vi "Configure Temperature Setpoint.vi"(8 "error in (no error)":errorcluster, 10 "Stirrer Speed Setpoint":dbl, 11 "heater_explorer in":refnum<class "heater_explorer.lvclass">) -> (0 "error out":errorcluster, 3 "heater_explorer out":refnum<class "heater_explorer.lvclass">)   [LabVIEW 2020, in "polar_bear_plus_drivers.lvlib" / "heater_explorer.lvclass"]
doc: "Changes the temperature setpoint."
uses:
  <instrlib>/RxnRover/Driver Polar Bear Plus/heater_explorer/heater_explorer.lvclass
  <instrlib>/RxnRover/Driver Polar Bear Plus/heater_explorer/heater_explorer.lvclass/heater_explorer.ctl
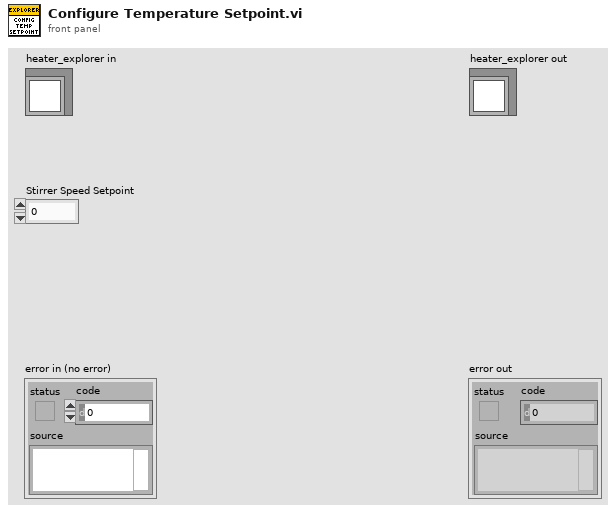
[diagram p1: front panel]
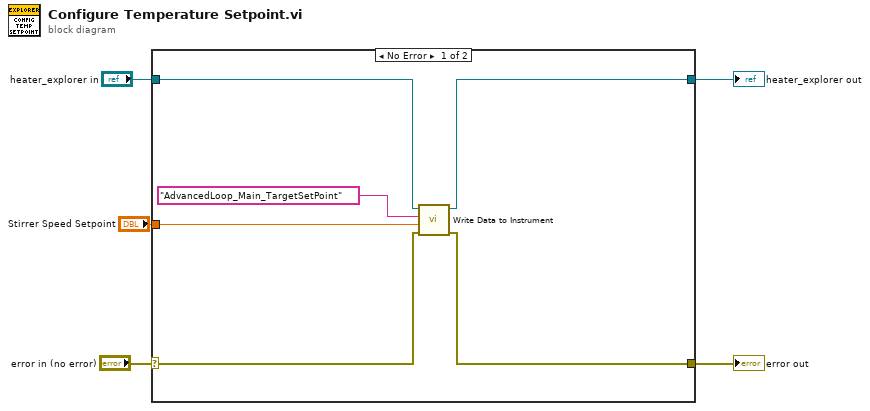
[diagram p0: block diagram]
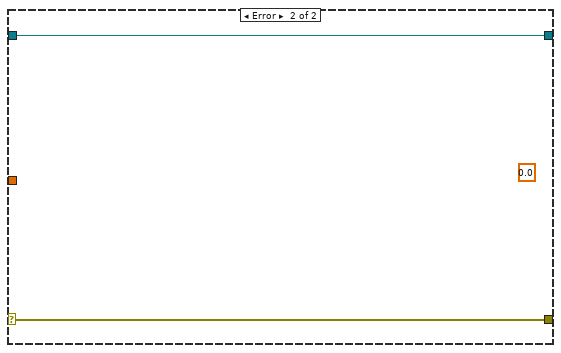
[diagram p2: hidden frame]
diagram:
  n1 = case shown="No Error" "error in (no error)" {
    selector: "error in (no error)" -> [w9 w12]
    tunnel: [w8 w12] -> w4
    tunnel: "heater_explorer in" -> [w11 w13]
    tunnel: [w10 w13] -> w2
    tunnel: "Stirrer Speed Setpoint" -> [w6 _]
    frame No Error {
      n2 = call-dynamic "Write Data to Instrument.vi"("error in (no error)"=w9, "Value to Send"=w6, "Address"="AdvancedLoop_Main_TargetSetPoint", "heater_parent in"=w11) -> ("error out"=w8:errorcluster, "heater_parent out"=w10:refnum<class "heater_explorer.lvclass">)  [unwired: 6 in]
    }
    frame Error {
      (unwired) 0.0 ("Value Read")
    }
  }
  "error out" <- w4
  "heater_explorer out" <- w2
